vi "2018版电磁铁-旋转.vi"(8 "速度选择":u16(ring)=1 items=["低速", "中速", "高速"], 9 "设定角度":dbl=1.0 format="%#_g°", 10 "方向选择":bool=TRUE, 11 "VISA资源名称":refnum<visa-resource-name>) -> ()   [LabVIEW 2019]
panel:
  in  "按钮":bool
  out "逆时针":bool
  out "顺时针":bool
  in  "驱动器细分":i16=10
  in  "转台减速比":dbl=496.0
  out "发送脉冲总数":u32
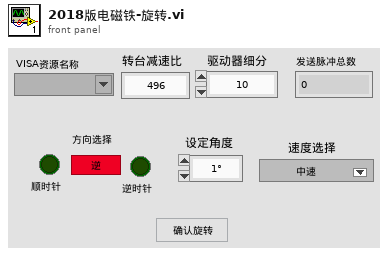
[diagram p1: front panel]
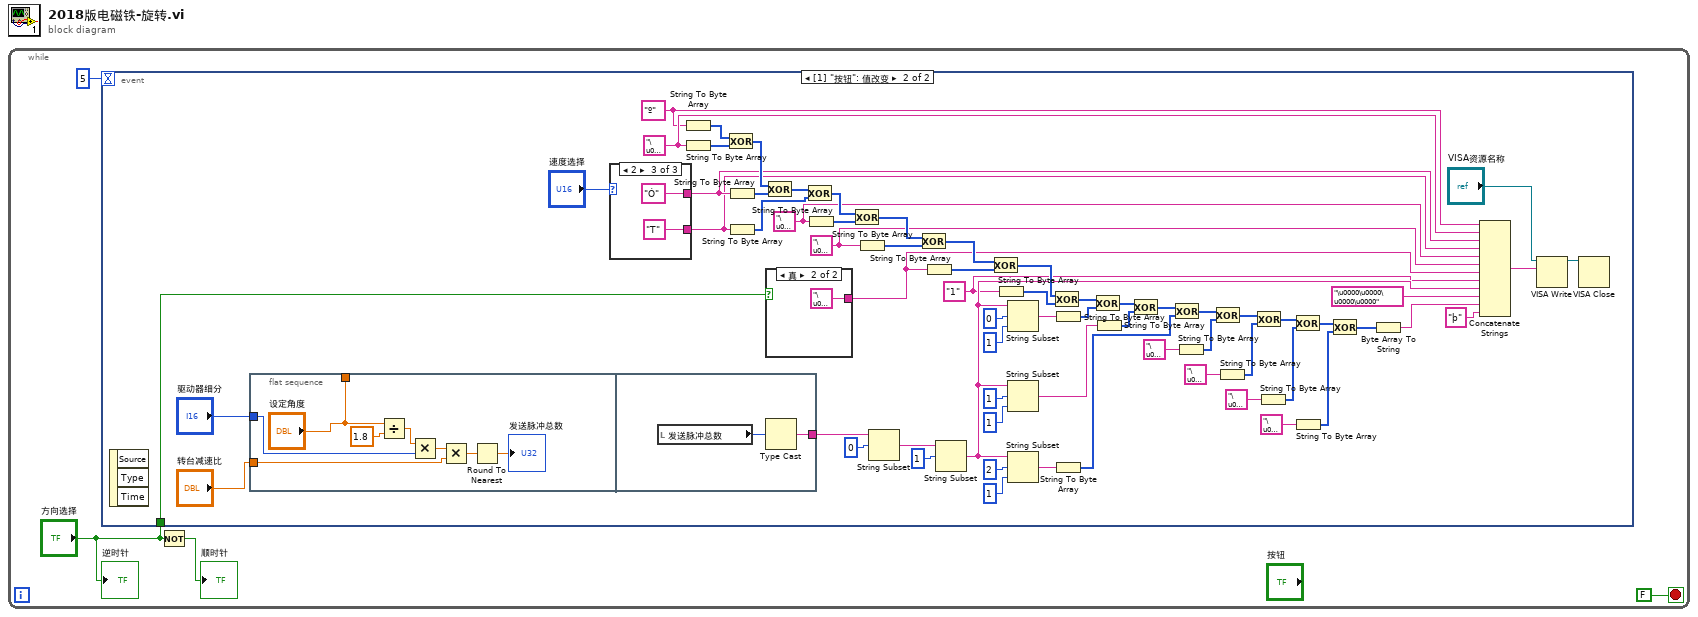
[diagram p0: block diagram]
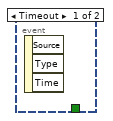
[diagram p2: hidden frame]
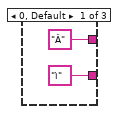
[diagram p3: hidden frame]
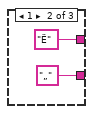
[diagram p4: hidden frame]
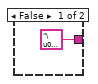
[diagram p5: hidden frame]
diagram:
  n1 = while {
    stop <- FALSE stop-if-true
    n2 = event shown="[1] \"按钮\": 值改变" {
      selector: _ -> [_ _]
      dyn-events: _ -> [_ _]
      timeout: 5 -> [_ _]
      tunnel: "方向选择" -> [_ w5]
      event Timeout {
        n3 = event-data() -> ()  [unwired: 1 in, 3 out]
      }
      event "按钮": Value Change {
        w13 = "\u0003"
        w14 = "1"
        w12 = "\u0000"
        w11 = "\u0001"
        w10 = "º"
        n4 = event-data() -> ()  [unwired: 1 in, 3 out]
        n5 = flat-sequence {
          tunnel: "驱动器细分" -> [w78]
          tunnel: "转台减速比" -> [w77]
          tunnel: ["设定角度"] -> _
          tunnel: [w84] -> w65
          frame #0 {
            n6 = Divide(x="设定角度", y=1.8) -> (x/y=w81:dbl)
            n7 = Multiply(x=w81, y=w78) -> (x*y=w82:dbl)
            n8 = Multiply(x=w82, y=w77) -> (x*y=w83:dbl)
            n9 = Round To Nearest(number=w83) -> (nearest integer value=→"发送脉冲总数":dbl)
          }
          frame #1 {
            n10 = local read "发送脉冲总数"() -> (w85:u32)
            n11 = Type Cast(x=w85) -> (*(type *) &x=w84:string)  [unwired: 1 in]
          }
        }
        n12 = case shown="2" "速度选择" {
          tunnel: ["ì" "„" "T"] -> w33
          tunnel: ["Â" "Ë" "Ó"] -> w34
          frame 0, Default {
          }
          frame 1 {
          }
          frame 2 {
          }
        }
        n13 = String To Byte Array(string=w10) -> (unsigned byte array=w63:u8[])
        n14 = String To Byte Array(string=w11) -> (unsigned byte array=w62:u8[])
        n15 = Exclusive Or(1:w62, 2:w63) -> (0:w58:u8[])
        n16 = String To Byte Array(string=w34) -> (unsigned byte array=w61:u8[])
        n17 = String To Byte Array(string=w33) -> (unsigned byte array=w60:u8[])
        n18 = Exclusive Or(1:w61, 2:w58) -> (0:w57:u8[])
        n19 = case shown="真" w5 {
          tunnel: ["\u0001" "\u0002"] -> w32
          frame False {
          }
          frame True {
          }
        }
        n20 = Exclusive Or(1:w60, 2:w57) -> (0:w56:u8[])
        n21 = String To Byte Array(string=w12) -> (unsigned byte array=w59:u8[])
        n22 = Exclusive Or(1:w59, 2:w56) -> (0:w55:u8[])
        n23 = String To Byte Array(string=w13) -> (unsigned byte array=w54:u8[])
        n24 = String Subset(string=w65, offset (0)=0) -> (substring=w66:string)  [unwired: 1 in]
        n25 = Exclusive Or(1:w54, 2:w55) -> (0:w53:u8[])
        n26 = String To Byte Array(string=w32) -> (unsigned byte array=w52:u8[])
        n27 = String Subset(string=w66, offset (0)=1) -> (substring=w30:string)  [unwired: 1 in]
        n28 = Exclusive Or(1:w52, 2:w53) -> (0:w51:u8[])
        n29 = String To Byte Array(string=w14) -> (unsigned byte array=w50:u8[])
        n30 = String Subset(string=w30, offset (0)=0, length (rest)=1) -> (substring=w29:string)
        n31 = String Subset(string=w30, offset (0)=1, length (rest)=1) -> (substring=w28:string)
        n32 = String Subset(string=w30, offset (0)=2, length (rest)=1) -> (substring=w27:string)
        n33 = Exclusive Or(1:w50, 2:w51) -> (0:w49:u8[])
        n34 = String To Byte Array(string=w29) -> (unsigned byte array=w48:u8[])
        n35 = String To Byte Array(string=w27) -> (unsigned byte array=w44:u8[])
        n36 = Exclusive Or(1:w48, 2:w49) -> (0:w47:u8[])
        n37 = String To Byte Array(string=w28) -> (unsigned byte array=w46:u8[])
        n38 = Exclusive Or(1:w46, 2:w47) -> (0:w45:u8[])
        n39 = Exclusive Or(1:w44, 2:w45) -> (0:w43:u8[])
        n40 = String To Byte Array(string="\u0000") -> (unsigned byte array=w42:u8[])
        n41 = Exclusive Or(1:w42, 2:w43) -> (0:w41:u8[])
        n42 = String To Byte Array(string="\u0000") -> (unsigned byte array=w40:u8[])
        n43 = Exclusive Or(1:w40, 2:w41) -> (0:w39:u8[])
        n44 = String To Byte Array(string="\u0000") -> (unsigned byte array=w38:u8[])
        n45 = Exclusive Or(1:w38, 2:w39) -> (0:w37:u8[])
        n46 = String To Byte Array(string="\u0000") -> (unsigned byte array=w36:u8[])
        n47 = Exclusive Or(1:w36, 2:w37) -> (0:w35:u8[])
        n48 = Byte Array To String(unsigned byte array=w35) -> (string=w31:string)
        n49 = Concatenate Strings(w10, w11, w34, w33, w12, w13, w32, w14, w30, "\u0000\u0000\u0000\u0000", w31, "þ") -> (w25:string)
        n50 = VISA Write(VISA resource name="VISA资源名称", write buffer=w25) -> (VISA resource name out=w26:refnum<visa-resource-name>)  [unwired: 1 in, 2 out]
        n51 = VISA Close(VISA resource name=w26) -> ()  [unwired: 1 in, 1 out]
      }
    }
    n52 = Not(x="方向选择") -> (.not. x?=→"顺时针":bool)
    "逆时针" <- "方向选择"
  }
